vi "Main.vi"(8 "error in":errorcluster, 11 "Status Platine Newport in":refnum<class "Status Platine Newport.lvclass">) -> (0 "error out":errorcluster, 3 "Status Platine Newport out":refnum<class "Status Platine Newport.lvclass">)   [LabVIEW 2024, in "Status Platine Newport.lvclass"]
doc: "The <b>Queued Message Handler</b> of the Worker that owns this VI."
uses:
  Status Platine Newport.lvclass
  Etat Status Platine.ctl
  Initialization Data.ctl
  Response Cases.ctl
  Status Platine Newport.lvclass/Status Platine Newport.ctl
  rql_Lecture Status en cours.ctl
  rqp_Start Status.ctl
  rqp_Stop Status.ctl
  Newport.SMC100.CommandInterface
  <vilib>/ErrorRing/Error Ring.xnode
panel:
  out "nombre (de 0 à 1)":dbl
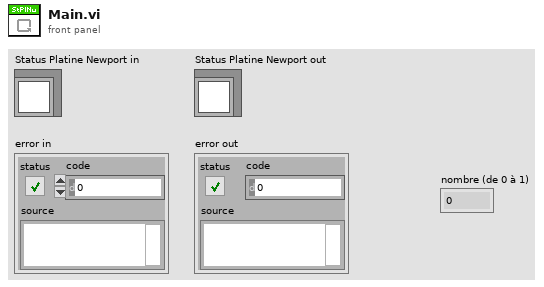
[diagram p1: front panel]
types:
  T1 = typedef "Status Platine Newport.lvclass/Etat Status Platine.ctl" = enum16{"Veille Status", "En Lecture Status", "Stop Stattus"}
  T2 = enum32{"Invalid", "Standard", "Closed", "Hidden", "Minimized", "Maximized"}
  T3 = typedef "Status Platine Newport.lvclass/Initialization Data.ctl" = cluster{"Response Cases":T4}
  T4 = typedef "Status Platine Newport.lvclass/Response Cases.ctl" = cluster{"Placeholder - Can be deleted":string, "SMC100 Reference":refnum<k24>, "RefnumStatus Platine":refnum<vi>}
  T5 = typedef "Status Platine Newport.lvclass/rql_Lecture Status en cours.ctl" = cluster{"String":string}
  T6 = typedef "Status Platine Newport.lvclass/rqp_Start Status.ctl" = cluster{"String":string, "RefnumStatus Platine":refnum<vi>}
  T7 = typedef "Status Platine Newport.lvclass/rqp_Stop Status.ctl" = cluster{"String":string}
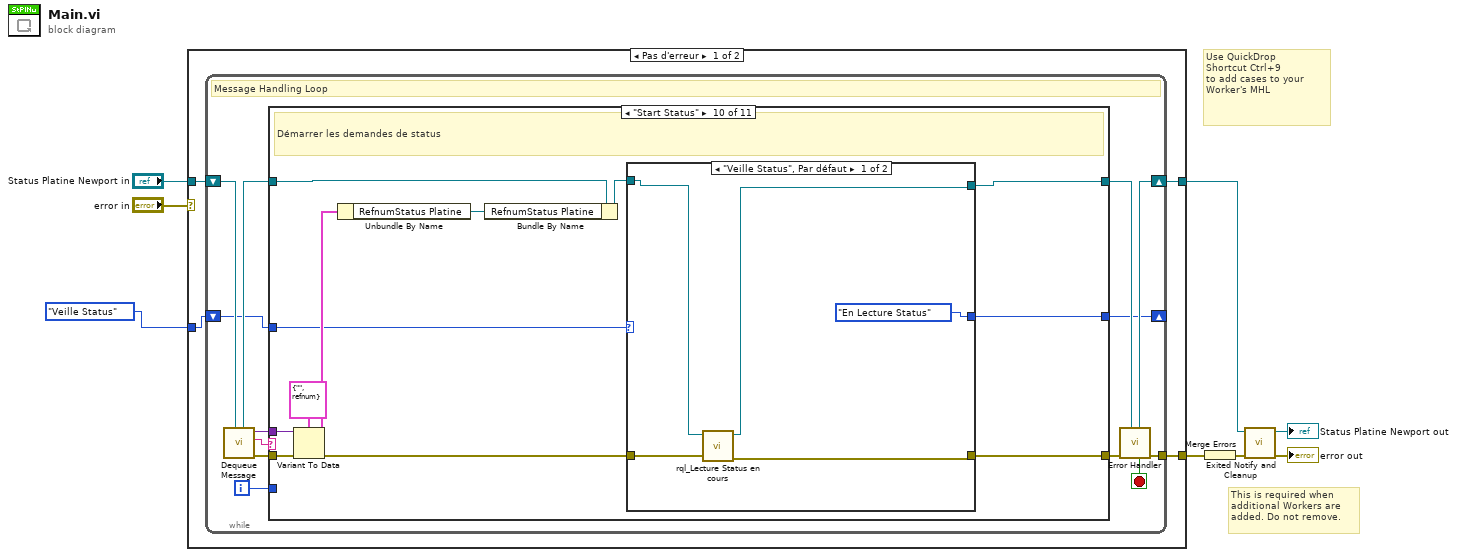
[diagram p0: block diagram]
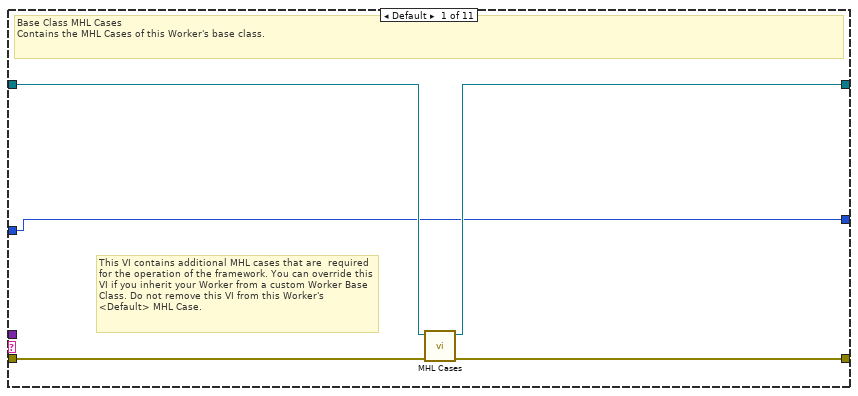
[diagram p2: hidden frame]
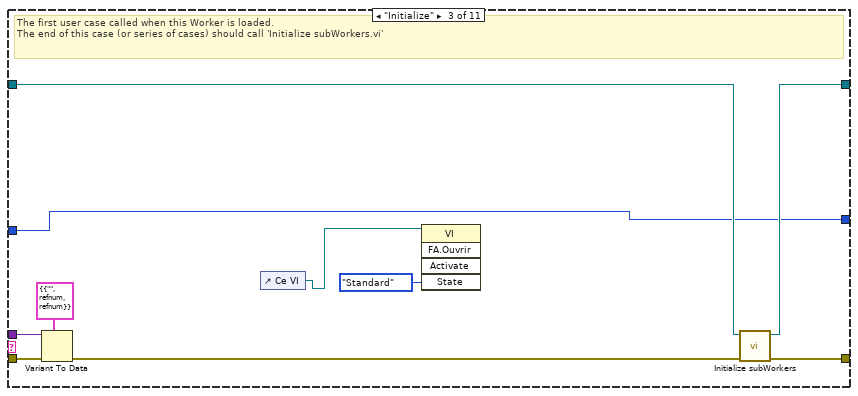
[diagram p4: hidden frame]
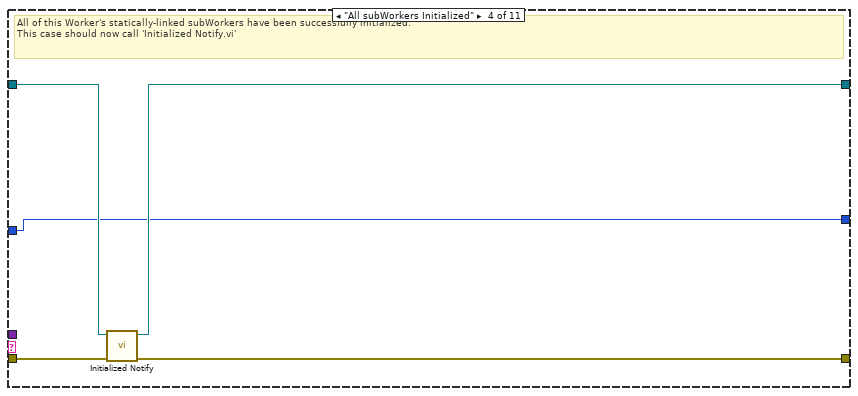
[diagram p5: hidden frame]
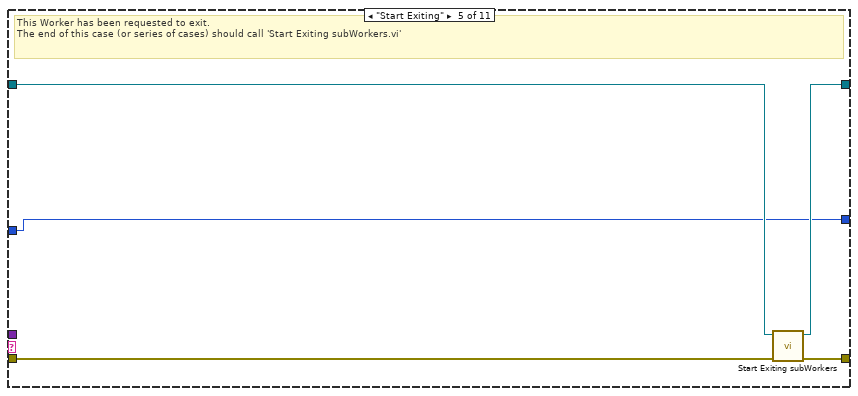
[diagram p6: hidden frame]
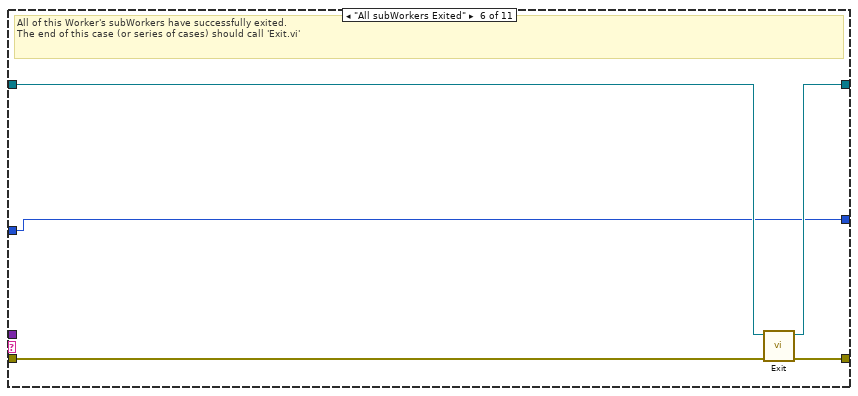
[diagram p7: hidden frame]
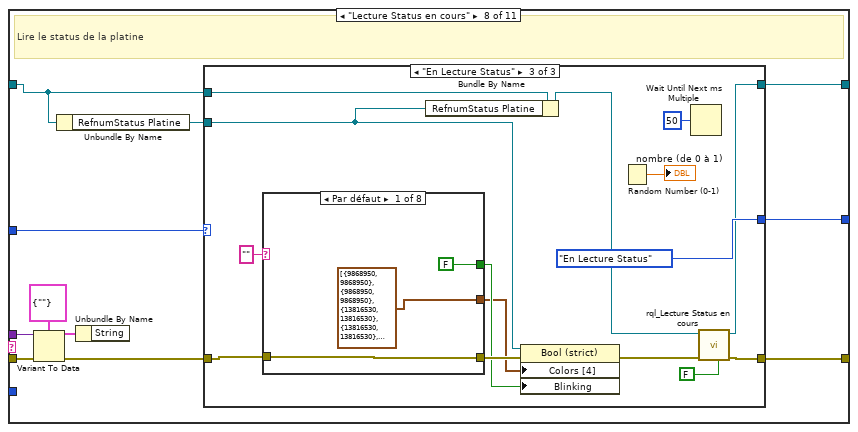
[diagram p9: hidden frame]
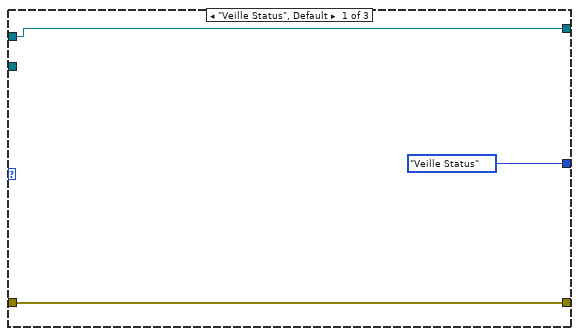
[diagram p10: hidden frame]
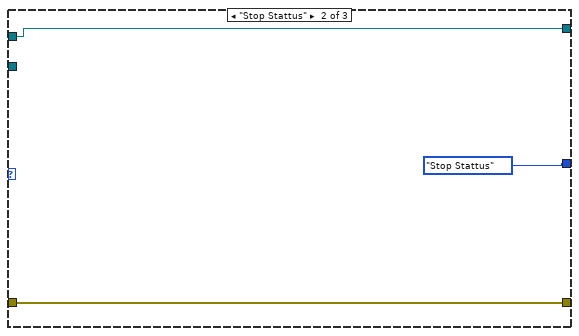
[diagram p11: hidden frame]
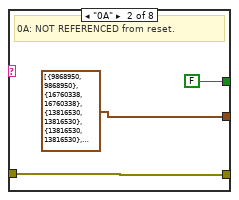
[diagram p12: hidden frame]
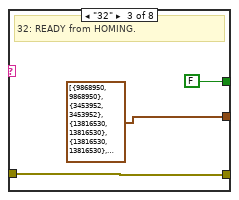
[diagram p13: hidden frame]
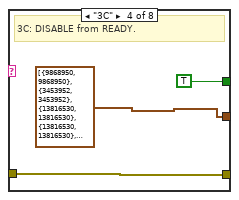
[diagram p14: hidden frame]
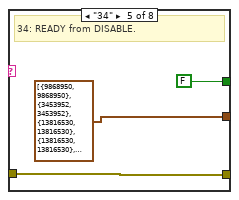
[diagram p15: hidden frame]
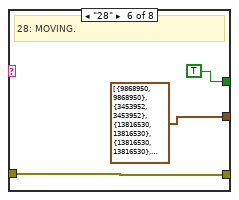
[diagram p16: hidden frame]
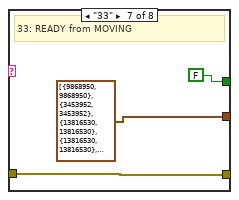
[diagram p17: hidden frame]
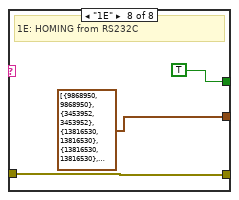
[diagram p18: hidden frame]
diagram:
  # "Use QuickDrop\nShortcut Ctrl+9\nto add cases to your\nWorker's MHL"
  # "This is required when additional Workers are added. Do not remove."
  n1 = case shown="Pas d'erreur" "error in" {
    tunnel: "Status Platine Newport in" -> [w10 w163]
    tunnel: [w12 w164] -> w7
    tunnel: [w11 w162] -> w8
    selector: "error in" -> [_ w165]
    tunnel: Etat_Status_Platine."Veille Status" ("Etat spectro") -> [w9 _]
    frame No Error {
      n2 = while {
        shift-right: [w23] -> w11
        shift-left: w10 -> [w25]
        tunnel: [w24] -> w12
        shift-right: [w14] -> _
        shift-left: w9 -> [w15]
        i -> [w16]
        stop <- w17 stop-if-true
        # "Message Handling Loop"
        n3 = call-dynamic "Dequeue Message.vi"("Worker"=w25) -> ("error out"=w22:errorcluster, "Case out"=w18:string, "Data out"=w13:variant, "Worker out"=w20:refnum<class "Status Platine Newport.lvclass">)  [unwired: 6 in, 1 out]
        n4 = case "Worker MHL Case Structure (DO NOT CHANGE LABEL NAME)" shown="\"Start Status\"" w18 {
          tunnel: w22 -> [w30 w32 w41 w48 w50 w58 w61 w72 w120 w132 w149]
          tunnel: [w29 w32 w43 w47 w53 w57 w61 w67 w120 w127 w144] -> w21
          tunnel: w20 -> [w28 w33 w40 w46 w51 w56 w60 w63 w119 w125 w142]
          tunnel: [w27 w33 w42 w45 w52 w55 w60 w65 w119 w126 w143] -> w19
          tunnel: w16 -> [_ _ _ _ _ _ _ _ _ _ _]
          tunnel: w15 -> [w26 w31 w34 w44 w49 w54 w59 w66 w118 w124 w141]
          tunnel: [w26 w31 w34 w44 w49 w54 w59 w64 w118 w123 w140] -> w14
          tunnel: w13 -> [_ _ w39 _ _ _ _ w69 _ w129 w146]
          frame Default {
            # "This VI contains additional MHL cases that are  required for the operation of the framework. You can override this VI if you inherit your Worker from a custom Worker Base Class. Do not remove this VI from this Worker's <Default> MHL Case."
            # "Base Class MHL Cases\nContains the MHL Cases of this Worker's base class."
            n5 = call-dynamic "MHL Cases.vi"("error in"=w30, "Worker in"=w28) -> ("error out"=w29:errorcluster, "Worker out"=w27:refnum<class "Status Platine Newport.lvclass">)  [unwired: 8 in]
          }
          frame "------------ FRAMEWORK CASES -----------" {
            # "Start of Workers Framework Cases"
          }
          frame "Initialize" {
            # "The first user case called when this Worker is loaded.\nThe end of this case (or series of cases) should call 'Initialize subWorkers.vi'"
            n6 = Variant To Data(error in=w41, type=T3 {"Response Cases"={"Placeholder - Can be deleted"="", "SMC100 Reference"=refnum, "RefnumStatus Platine"=refnum}} ("Cluster"), Variant=w39) -> (error out=w35:errorcluster)  [unwired: 1 out]
            n7 = control-ref of="Ce VI"() -> (w37:refnum<vi>)
            n8 = invoke class="VI" method="FA.Ouvrir"(reference=w37, "State"=T2."Standard" ("État")) -> ()  [unwired: 3 in, 5 out]
            n9 = call-dynamic "Initialize subWorkers.vi"("error in"=w35, "Worker"=w40) -> ("error out"=w43:errorcluster, "dup Worker out"=w42:refnum<class "Status Platine Newport.lvclass">)  [unwired: 8 in]
          }
          frame "All subWorkers Initialized" {
            # "All of this Worker's statically-linked subWorkers have been successfully initialized.\nThis case should now call 'Initialized Notify.vi'"
            n10 = call-dynamic "Initialized Notify.vi"("error in"=w48, "Worker"=w46) -> ("error out"=w47:errorcluster, "dup Worker out"=w45:refnum<class "Status Platine Newport.lvclass">)  [unwired: 8 in]
          }
          frame "Start Exiting" {
            # "This Worker has been requested to exit. \nThe end of this case (or series of cases) should call 'Start Exiting subWorkers.vi'"
            n11 = call-dynamic "Start Exiting subWorkers.vi"("error_in"=w50, "Worker"=w51) -> ("error out"=w53:errorcluster, "dup Worker out"=w52:refnum<class "Status Platine Newport.lvclass">)  [unwired: 8 in]
          }
          frame "All subWorkers Exited" {
            # "All of this Worker's subWorkers have successfully exited. \nThe end of this case (or series of cases) should call 'Exit.vi'"
            n12 = call-dynamic "Exit.vi"("error_in"=w58, "Worker"=w56) -> ("error out"=w57:errorcluster, "dup Worker out"=w55:refnum<class "Status Platine Newport.lvclass">)  [unwired: 8 in]
          }
          frame "------------- LOCAL API CASES -------------" {
            # "Start of Workers Local API Cases"
          }
          frame "Lecture Status en cours" {
            # "Lire le status de la platine"
            n13 = Variant To Data(error in=w72, type=T5 {"String"=""} ("Data"), Variant=w69) -> (data=w68:T5, error out=w71:errorcluster)
            n14 = Unbundle By Name(w63) -> ("RefnumStatus Platine"=w62:refnum<vi>)
            n15 = Unbundle By Name(w68) -> ()  [unwired: 1 out]
            n16 = case shown="\"En Lecture Status\"" w66 {
              tunnel: w71 -> [w74 w78 w86]
              tunnel: [w74 w78 w90] -> w67
              tunnel: [w75 w77 w88] -> w65
              tunnel: w63 -> [w75 w77 w89]
              tunnel: [Etat_Status_Platine."Veille Status" ("Etat spectro") Etat_Status_Platine."Stop Stattus" ("Etat spectro") Etat_Status_Platine."En Lecture Status" ("Etat spectro")] -> w64
              tunnel: w62 -> [_ _ w79]
              frame "Veille Status", Default {
              }
              frame "Stop Stattus" {
              }
              frame "En Lecture Status" {
                n17 = case shown="Par défaut" "" {
                  tunnel: w86 -> [w96 w99 w102 w105 w108 w111 w114 w117]
                  tunnel: [w96 w99 w102 w105 w108 w111 w114 w117] -> w84
                  tunnel: [cluster{u32, u32}[] [{9868950, 9868950}, {9868950, 9868950}, {13816530, 13816530}, {13816530, 13816530}, {16777216, 16777216}, {16777216, 16777216}] cluster{u32, u32}[] [{9868950, 9868950}, {16760338, 16760338}, {13816530, 13816530}, {13816530, 13816530}, {16777216, 16777216}, {16777216, 16777216}] cluster{u32, u32}[] [{9868950, 9868950}, {3453952, 3453952}, {13816530, 13816530}, {13816530, 13816530}, {16777216, 16777216}, {16777216, 16777216}] cluster{u32, u32}[] [{9868950, 9868950}, {3453952, 3453952}, {13816530, 13816530}, {13816530, 13816530}, {16777216, 16777216}, {16777216, 16777216}] cluster{u32, u32}[] [{9868950, 9868950}, {3453952, 3453952}, {13816530, 13816530}, {13816530, 13816530}, {16777216, 16777216}, {16777216, 16777216}] cluster{u32, u32}[] [{9868950, 9868950}, {3453952, 3453952}, {13816530, 13816530}, {13816530, 13816530}, {16777216, 16777216}, {16777216, 16777216}] cluster{u32, u32}[] [{9868950, 9868950}, {3453952, 3453952}, {13816530, 13816530}, {13816530, 13816530}, {16777216, 16777216}, {16777216, 16777216}] cluster{u32, u32}[] [{9868950, 9868950}, {3453952, 3453952}, {13816530, 13816530}, {13816530, 13816530}, {16777216, 16777216}, {16777216, 16777216}]] -> w81
                  tunnel: [FALSE FALSE FALSE TRUE FALSE TRUE FALSE TRUE] -> w82
                  frame Default {
                  }
                  frame "0A" {
                    # "0A: NOT REFERENCED from reset."
                  }
                  frame "32" {
                    # "32: READY from HOMING."
                  }
                  frame "3C" {
                    # "3C: DISABLE from READY."
                  }
                  frame "34" {
                    # "34: READY from DISABLE."
                  }
                  frame "28" {
                    # "28: MOVING."
                  }
                  frame "33" {
                    # "33: READY from MOVING"
                  }
                  frame "1E" {
                    # "1E: HOMING from RS232C"
                  }
                }
                n18 = Bundle By Name(cluster=w89, "RefnumStatus Platine"=w79) -> (w80:refnum<class "Status Platine Newport.lvclass">)
                n19 = property class="Bool (strict)"(reference=w79, error in=w84, "Colors [4]"=w81, "Blinking"=w82) -> (error out=w83:errorcluster)  [unwired: 1 out]
                n20 = Random Number (0-1)() -> (number: 0 to 1=→"nombre (de 0 à 1)":dbl)
                n21 = Wait Until Next ms Multiple(millisecond multiple=u32 50 ("attente (ms)")) -> ()  [unwired: 1 out]
                n22 = call "rql_Lecture Status en cours.vi"("Show in Debugger?"=FALSE, "error in"=w83, "Status Platine Newport in"=w80) -> ("error out"=w90:errorcluster, "dup Status Platine Newport out"=w88:refnum<class "Status Platine Newport.lvclass">)  [unwired: 7 in]
              }
            }
          }
          frame "------------- PUBLIC API CASES -------------" {
            # "Start of Workers Public API Cases"
          }
          frame "Start Status" {
            # "Démarrer les demandes de status"
            n23 = Variant To Data(error in=w132, type=T6 {"String"="", "RefnumStatus Platine"=refnum} ("Data"), Variant=w129) -> (data=w128:T6, error out=w131:errorcluster)
            n24 = Unbundle By Name(w128) -> ("RefnumStatus Platine"=w121:refnum<vi>)
            n25 = Bundle By Name(cluster=w125, "RefnumStatus Platine"=w121) -> (w122:refnum<class "Status Platine Newport.lvclass">)
            n26 = case shown="\"Veille Status\", Par défaut" w124 {
              tunnel: w131 -> [w136 w139]
              tunnel: [w135 w139] -> w127
              tunnel: [w133 w138] -> w126
              tunnel: w122 -> [w134 w138]
              tunnel: [Etat_Status_Platine."En Lecture Status" ("Etat spectro") _] -> w123
              frame "Veille Status", Default {
                n27 = call "rql_Lecture Status en cours.vi"("error in"=w136, "Status Platine Newport in"=w134) -> ("error out"=w135:errorcluster, "dup Status Platine Newport out"=w133:refnum<class "Status Platine Newport.lvclass">)  [unwired: 8 in]
              }
              frame "En Lecture Status" {
              }
            }
          }
          frame "Stop Status" {
            # "Arrête la lecture du status de la platine"
            n28 = Variant To Data(error in=w149, type=T7 {"String"=""} ("Data"), Variant=w146) -> (data=w145:T7, error out=w148:errorcluster)
            n29 = Unbundle By Name(w145) -> ()  [unwired: 1 out]
            n30 = case shown="\"Veille Status\", Par défaut" w141 {
              tunnel: w148 -> [w152 w155 w160]
              tunnel: [w152 w155 w159] -> w144
              tunnel: [w151 w154 w157] -> w143
              tunnel: w142 -> [w151 w154 w157]
              tunnel: [Etat_Status_Platine."Veille Status" ("Etat spectro") Etat_Status_Platine."Veille Status" ("Etat spectro") Etat_Status_Platine."Stop Stattus" ("Etat spectro")] -> w140
              frame "Veille Status", Default {
              }
              frame "Stop Stattus" {
              }
              frame "En Lecture Status" {
                n31 = xnode ("Error_Ring")() -> ("sortie d'erreur"=w158:errorcluster)
                n32 = Merge Errors(w160, w158) -> (w159:errorcluster)
              }
            }
          }
        }
        n33 = call-dynamic "Error Handler.vi"("Worker"=w19, "error_in"=w21) -> ("error out"=w24:errorcluster, "Stop Loop"=w17:bool, "Worker out"=w23:refnum<class "Status Platine Newport.lvclass">)  [unwired: 7 in]
      }
    }
    frame Error {
      n34 = call-dynamic "Error Handler.vi"("Worker"=w163, "error_in"=w165) -> ("error out"=w164:errorcluster, "Worker out"=w162:refnum<class "Status Platine Newport.lvclass">)  [unwired: 7 in, 1 out]
    }
  }
  n35 = Merge Errors(w7) -> (w4:errorcluster)
  n36 = call-dynamic "Exited Notify and Cleanup.vi"("error_in"=w4, "Worker"=w8) -> ("error out"=→"error out":errorcluster, "dup Worker out"=→"Status Platine Newport out":refnum<class "Status Platine Newport.lvclass">)  [unwired: 8 in]
